vi "Full Real Matrix Cholesky Factorization.vi"(0 "A":T1) -> (1 "Cholesky":T1, 2 "error":i32)   [LabVIEW 2020, in "NI_AALBase.lvlib"]
doc: "Cholesky decompostion: input and output matrix both in full storage"
uses:
  <vilib>/Analysis/NI_AALBase.lvlib
  <vilib>/Analysis/Matrix/Datatypes/RealMatrix.ctl
  <resource>/lvanlys.dll
  <vilib>/Analysis/Matrix/NI_Matrix.lvlib
panel:
  # "Full Matrix Cholesky Factorization"
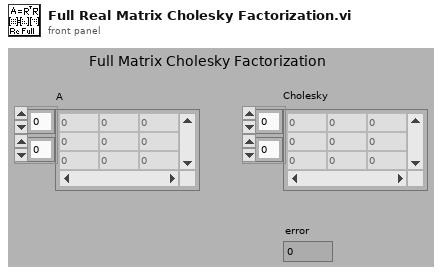
[diagram p1: front panel]
types:
  T1 = typedef "NI_Matrix.lvlib/RealMatrix.ctl" = dbl[][]
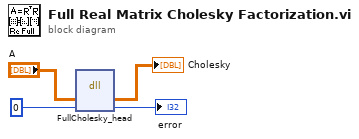
[diagram p0: block diagram]
diagram:
  n1 = dll-call lib="e:/builds/penguin/labview/branches/2020/dev/dist/resource/lvanlys.*" fn="FullCholesky_head"("A"="A", "error"=0) -> ("A"=→"Cholesky":T1, "error"=→"error":i32)  [unwired: 4 in, 2 out]
